vi "RF Offset.vi"() -> ()   [LabVIEW 2018]
uses:
  <vilib>/Analysis/baseanly.llb/Mean (DBL).vi
  <vilib>/express/express shared/transition.llb/Dynamic To Waveform Array.vi
  <vilib>/express/express signal manip/GetorSetDDTAttributes/Set DDT Attributes/SetT0.vi
  <vilib>/express/express shared/transition.llb/Waveform Array To Dynamic.vi
  <vilib>/express/express signal manip/GetorSetDDTAttributes/Set DDT Attributes/Set DDT Properties.xnode
  <vilib>/Analysis/NI_AALBase.lvlib
panel:
  out "Filename Out":path
  in  "Filename":path=path "C:/Users/physics-svc-fulda/Desktop/LabVIEW Data/RF OFFset.lvm"
  out "Waveform Graph":dynamicdata(graph)
  out "Saving Data":bool
  in  "Enable":bool=TRUE
  out "RF D":dbl format="%0.6f"
  out "RF C":dbl format="%0.6f"
  out "RF B":dbl format="%0.6f"
  out "RF A":dbl format="%0.6f"
  in  "timeout (s)":dbl=10.0 format="%0.2f"
  in  "rate":dbl=1000.0
  in  "# of samples":i32=100
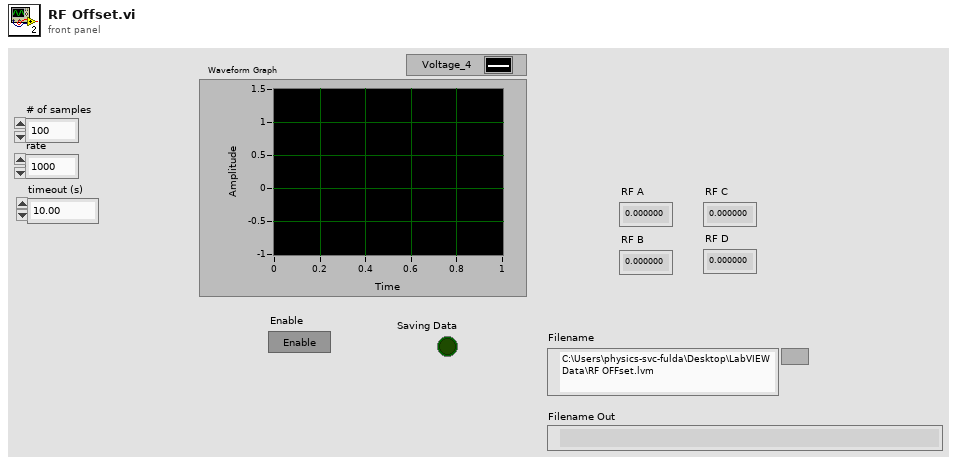
[diagram p1: front panel]
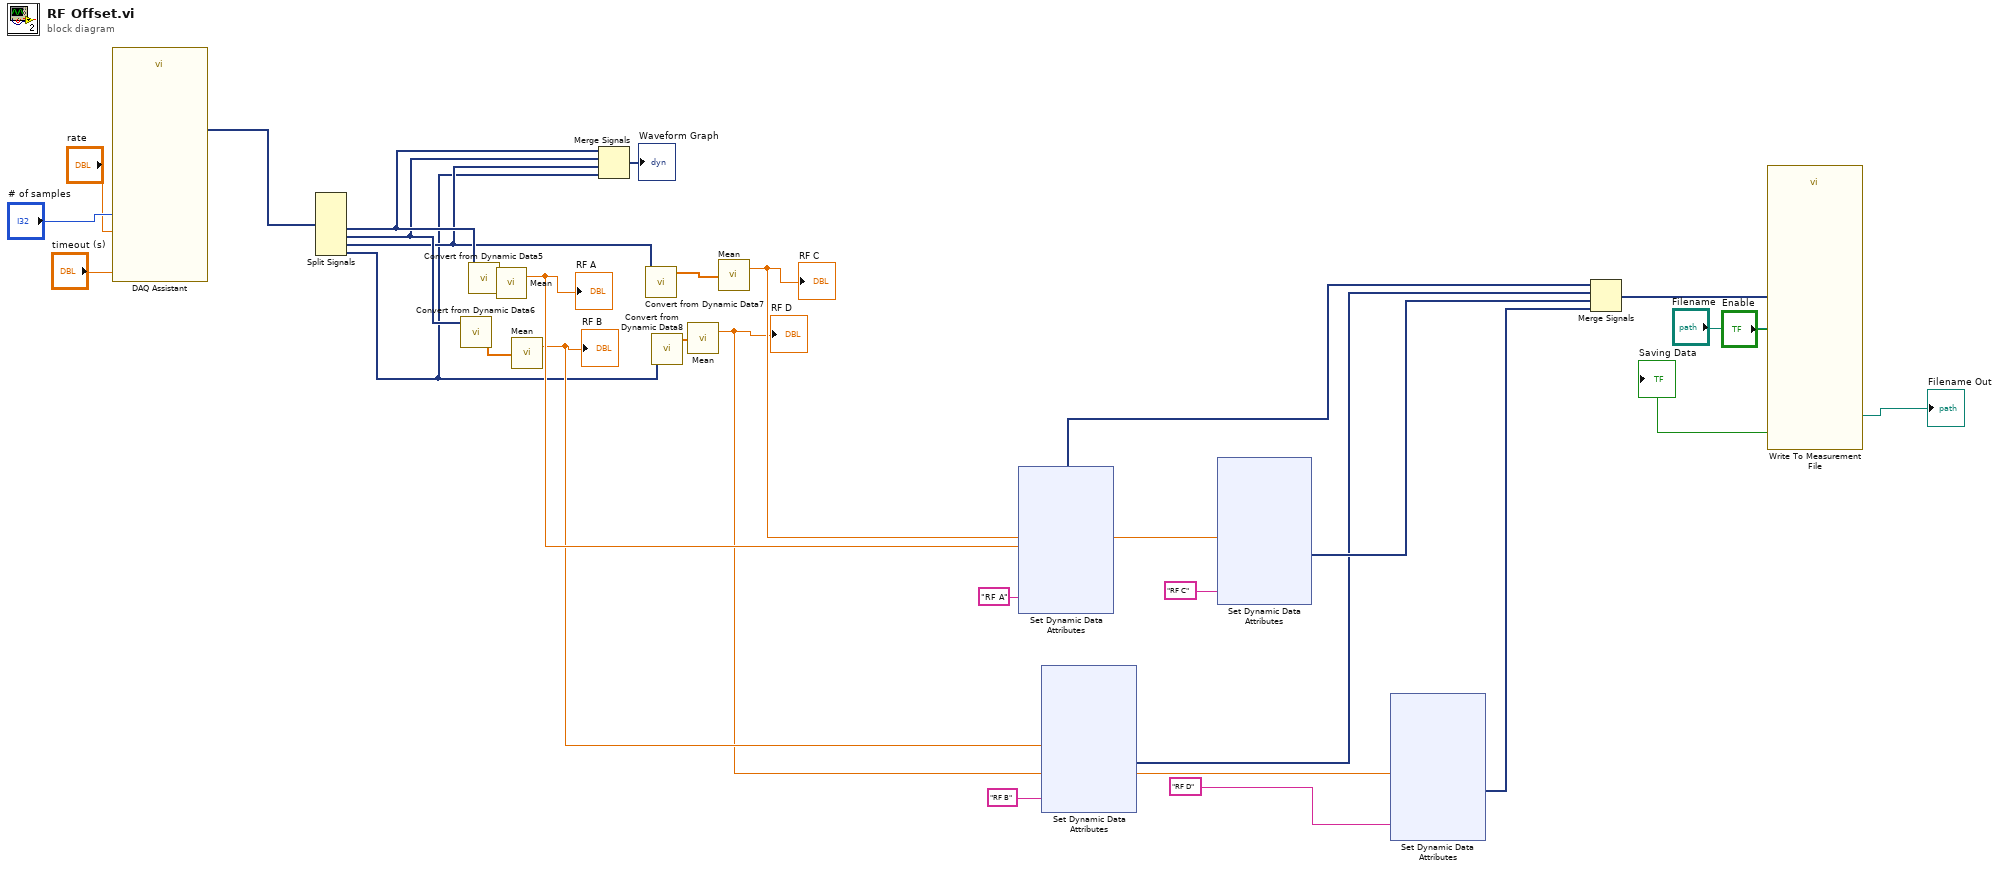
[diagram p0: block diagram]
diagram:
  n1 = call "DAQ Assistant"("rate"="rate", "number of samples"="# of samples", "timeout (s)"="timeout (s)") -> ("data"=w27:dynamicdata)  [unwired: 14 in, 2 out]
  n2 = Split Signals(w27) -> (w7:dynamicdata, w6:dynamicdata, w5:dynamicdata, w4:dynamicdata)  [unwired: 8 in, 4 out]
  n3 = call "Convert from Dynamic Data6"("Dynamic Data Type"=w6) -> ("Array"=w25:dbl[])  [unwired: 3 in]
  n4 = call "Convert from Dynamic Data5"("Dynamic Data Type"=w7) -> ("Array"=w26:dbl[])  [unwired: 3 in]
  n5 = call-poly <vilib>:"Mean.vi"("X"=w26) -> ("mean"=w19:dbl)  [unwired: 1 out]
  "RF A" <- w19
  n6 = call-poly <vilib>:"Mean.vi"("X"=w25) -> ("mean"=w18:dbl)  [unwired: 1 out]
  "RF B" <- w18
  n7 = Merge Signals(w7, w6, w5, w4) -> (→"Waveform Graph":dynamicdata)
  n8 = call "Convert from Dynamic Data7"("Dynamic Data Type"=w5) -> ("Array"=w24:dbl[])  [unwired: 3 in]
  n9 = call "Convert from Dynamic Data8"("Dynamic Data Type"=w4) -> ("Array"=w23:dbl[])  [unwired: 3 in]
  n10 = call-poly <vilib>:"Mean.vi"("X"=w23) -> ("mean"=w16:dbl)  [unwired: 1 out]
  "RF D" <- w16
  n11 = call-poly <vilib>:"Mean.vi"("X"=w24) -> ("mean"=w17:dbl)  [unwired: 1 out]
  "RF C" <- w17
  n12 = xnode "Set Dynamic Data Attributes"("Signals In"=w19, "Signal Name"="RF A") -> ("Signals Out"=w11:dynamicdata)  [unwired: 2 in, 1 out]
  n13 = xnode "Set Dynamic Data Attributes"("Signals In"=w18, "Signal Name"="RF B") -> ("Signals Out"=w9:dynamicdata)  [unwired: 2 in, 1 out]
  n14 = xnode "Set Dynamic Data Attributes"("Signals In"=w17, "Signal Name"="RF C") -> ("Signals Out"=w10:dynamicdata)  [unwired: 2 in, 1 out]
  n15 = xnode "Set Dynamic Data Attributes"("Signals In"=w16, "Signal Name"="RF D") -> ("Signals Out"=w8:dynamicdata)  [unwired: 2 in, 1 out]
  n16 = Merge Signals(w11, w9, w10, w8) -> (w22:dynamicdata)
  n17 = call "Write To Measurement File"("Signals"=w22, "Enable"="Enable", "Filename"="Filename") -> ("Filename Out"=→"Filename Out":path, "Saving Data"=→"Saving Data":bool)  [unwired: 14 in, 1 out]
